vi "log analysis_gps.vi"() -> ()   [LabVIEW 2019] (continued)
-0.0020,-0.483216711,-1.218552457,32.463260828,0.4082,0.2863,0.5249,0.1204,0.1022,0.0792,0.2990,0.3004,4.9651,0f000001,0*7877b410\n\t", "INSPVAXA,USB3,0,45.5,FINESTEERING,2107,281168.650,02000000,471d,15824;INS_ALIGNMENT_COMPLETE,INS_RTKFIXED,37.37019633744,126.72089858847,9.9020,22.3000,0.4572,0.3119,0.0094,-0.439520835,-0.957492339,36.615351128,0.4109,0.2881,0.5277,0.1190,0.0994,0.0787,0.2969,0.2961,4.9653,0f000001,0*c67ea19b\n\t", "INSPVAXA,USB3,0,41.5,FINESTEERING,2107,281169.150,02000000,471d,15824;INS_ALIGNMENT_COMPLETE,INS_RTKFIXED,37.37019803366,126.72090033617,9.8967,22.3000,0.4353,0.3466,-0.0124,-0.373798304,-0.691045943,38.520831977,0.4135,0.2910,0.5324,0.1162,0.0959,0.0784,0.2944,0.2920,4.9653,0f000001,0*85acc37f\n\t", "INSPVAXA,USB3,0,41.5,FINESTEERING,2107,281169.650,02000000,471d,15824;INS_ALIGNMENT_COMPLETE,INS_RTKFIXED,37.37019968370,126.72090219115,9.8910,22.3000,0.4092,0.3296,-0.0191,-0.608129529,-0.998598974,40.257706862,0.4135,0.2910,0.5324,0.1162,0.0959,0.0784,0.2944,0.2920,4.9653,0f000001,0*4e1130ac\n\t", "INSPVAXA,USB3,0,45.5,FINESTEERING,2107,281170.150,02000000,471d,15824;INS_ALIGNMENT_COMPLETE,INS_RTKFIXED,37.37020123427,126.72090408580,9.8830,22.3000,0.3824,0.3449,-0.0045,-0.472006885,-0.997512763,41.710684669,0.4139,0.2909,0.5351,0.1136,0.0932,0.0791,0.2920,0.2885,4.9641,0f000001,0*2dc0ad9b\n\t", "INSPVAXA,USB3,0,45.5,FINESTEERING,2107,281170.650,02000000,471d,15824;INS_ALIGNMENT_COMPLETE,INS_RTKFIXED,37.37020269712,126.72090601410,9.8764,22.3000,0.3826,0.3439,-0.0555,-0.519783559,-1.040179137,42.895943819,0.4139,0.2909,0.5351,0.1136,0.0932,0.0791,0.2920,0.2885,4.9641,0f000001,0*7bedead2\n\t", "INSPVAXA,USB3,0,44.5,FINESTEERING,2107,281171.150,02000000,471d,15824;INS_ALIGNMENT_COMPLETE,INS_RTKFIXED,37.37020410008,126.72090794331,9.8693,22.3000,0.3861,0.3636,0.0003,-0.699793085,-1.013428627,43.781952509,0.4138,0.2914,0.5397,0.1111,0.0916,0.0789,0.2901,0.2864,4.9621,0f000001,0*75d8a529\n\t", "INSPVAXA,USB3,0,44.5,FINESTEERING,2107,281171.650,02000000,471d,15824;INS_ALIGNMENT_COMPLETE,INS_RTKFIXED,37.37020547941,126.72090993032,9.8591,22.3000,0.3712,0.3482,-0.0204,-0.626506310,-1.371933495,44.325085685,0.4138,0.2914,0.5397,0.1111,0.0916,0.0789,0.2901,0.2864,4.9621,0f000001,0*603a8c7d\n\t", "INSPVAXA,USB3,0,46.5,FINESTEERING,2107,281172.150,02000000,471d,15824;INS_ALIGNMENT_COMPLETE,INS_RTKFIXED,37.37020680132,126.72091185634,9.8504,22.3000,0.3423,0.3408,-0.0083,-0.892607382,-1.242115699,44.703288237,0.4137,0.2941,0.5475,0.1101,0.0921,0.0790,0.2889,0.2855,4.9595,0f000001,0*90544be8\n\t", "INSPVAXA,USB3,0,46.5,FINESTEERING,2107,281172.650,02000000,471d,15824;INS_ALIGNMENT_COMPLETE,INS_RTKFIXED,37.37020806274,126.72091379412,9.8428,22.3000,0.3393,0.3608,-0.0229,-0.508945363,-1.293654987,44.950159425,0.4137,0.2941,0.5475,0.1101,0.0921,0.0790,0.2889,0.2855,4.9595,0f000001,0*b56eb890\n\t", "INSPVAXA,USB3,0,45.0,FINESTEERING,2107,281173.150,02000000,471d,15824;INS_ALIGNMENT_COMPLETE,INS_RTKFIXED,37.37020938618,126.72091581251,9.8332,22.3000,0.3324,0.3645,-0.0096,-0.521372580,-0.940346469,45.114108155,0.4131,0.2953,0.5536,0.1104,0.0943,0.0789,0.2883,0.2853,4.9566,0f000001,0*896df924\n\t", "INSPVAXA,USB3,0,45.0,FINESTEERING,2107,281173.650,02000000,471d,15824;INS_ALIGNMENT_COMPLETE,INS_RTKFIXED,37.37021062105,126.72091771518,9.8279,22.3000,0.3141,0.3794,-0.0018,-0.763185421,-1.256731125,45.193767644,0.4131,0.2953,0.5536,0.1104,0.0943,0.0789,0.2883,0.2853,4.9566,0f000001,0*bce21ee6\n\t", "INSPVAXA,USB3,0,42.5,FINESTEERING,2107,281174.150,02000000,471d,15824;INS_ALIGNMENT_COMPLETE,INS_RTKFIXED,37.37021196803,126.72091978453,9.8240,22.3000,0.3107,0.3301,0.0022,-0.763032701,-1.186677441,45.109324656,0.4135,0.2997,0.5622,0.1120,0.0966,0.0795,0.2881,0.2853,4.9521,0f000001,0*4885d5cd\n\t", "INSPVAXA,USB3,0,42.5,FINESTEERING,2107,281174.650,02000000,471d,15824;INS_ALIGNMENT_COMPLETE,INS_RTKFIXED,37.37021324009,126.72092171742,9.8181,22.3000,0.3189,0.3639,-0.0177,-0.623768140,-1.260059850,44.385500285,0.4135,0.2997,0.5622,0.1120,0.0966,0.0795,0.2881,0.2853,4.9521,0f000001,0*5d7db614\n\t", "INSPVAXA,USB3,0,46.0,FINESTEERING,2107,281175.150,02000000,471d,15824;INS_ALIGNMENT_COMPLETE,INS_RTKFIXED,37.37021454485,126.72092359431,9.8111,22.3000,0.2994,0.3285,-0.0007,-0.912779431,-1.090246712,43.056876175,0.4145,0.3032,0.5695,0.1139,0.0990,0.0803,0.2881,0.2850,4.9479,0f000001,0*1b591d65\n\t", "INSPVAXA,USB3,0,46.0,FINESTEERING,2107,281175.650,02000000,471d,15824;INS_ALIGNMENT_COMPLETE,INS_RTKFIXED,37.37021589583,126.72092544139,9.8034,22.3000,0.3183,0.3129,-0.0016,-0.983600306,-1.421345156,41.411365334,0.4145,0.3032,0.5695,0.1139,0.0990,0.0803,0.2881,0.2850,4.9479,0f000001,0*27aaa3ef\n\t", "INSPVAXA,USB3,0,44.5,FINESTEERING,2107,281176.150,02000000,471d,15824;INS_ALIGNMENT_COMPLETE,INS_RTKFIXED,37.37021731136,126.72092726471,9.7967,22.3000,0.3067,0.3205,0.0018,-0.778712195,-1.421988866,39.539976805,0.4163,0.3059,0.5758,0.1149,0.0990,0.0812,0.2880,0.2842,4.9430,0f000001,0*48a96dd4\n\t", "INSPVAXA,USB3,0,44.5,FINESTEERING,2107,281176.650,02000000,471d,15824;INS_ALIGNMENT_COMPLETE,INS_RTKFIXED,37.37021874043,126.72092900172,9.7912,22.3000,0.3343,0.3105,-0.0118,-0.475424413,-1.033048404,37.733219685,0.4163,0.3059,0.5758,0.1149,0.0990,0.0812,0.2880,0.2842,4.9430,0f000001,0*63ca753e\n\t", "INSPVAXA,USB3,0,46.0,FINESTEERING,2107,281177.150,02000000,471d,15824;INS_ALIGNMENT_COMPLETE,INS_RTKFIXED,37.37022027462,126.72093069920,9.7837,22.3000,0.3340,0.3056,-0.0059,-0.436029262,-1.318996825,36.094424232,0.4169,0.3052,0.5779,0.1146,0.0975,0.0816,0.2876,0.2828,4.9395,0f000001,0*8ee0afa4\n\t", "INSPVAXA,USB3,0,46.0,FINESTEERING,2107,281177.650,02000000,471d,15824;INS_ALIGNMENT_COMPLETE,INS_RTKFIXED,37.37022187937,126.72093233106,9.7786,22.3000,0.3383,0.3047,-0.0171,-0.416097585,-1.463260618,34.652814665,0.4169,0.3052,0.5779,0.1146,0.0975,0.0816,0.2876,0.2828,4.9395,0f000001,0*8906ebb7\n\t", "INSPVAXA,USB3,0,43.5,FINESTEERING,2107,281178.150,02000000,471d,15824;INS_ALIGNMENT_COMPLETE,INS_RTKFIXED,37.37022350567,126.72093390601,9.7761,22.3000,0.3475,0.2828,-0.0164,-0.206861779,-1.246508732,33.446442474,0.4170,0.3028,0.5771,0.1137,0.0954,0.0819,0.2871,0.2813,4.9371,0f000001,0*562de2ee\n\t", "INSPVAXA,USB3,0,43.5,FINESTEERING,2107,281178.650,02000000,471d,15824;INS_ALIGNMENT_COMPLETE,INS_RTKFIXED,37.37022519841,126.72093545972,9.7722,22.3000,0.3782,0.2868,-0.0191,-0.115839581,-1.073328137,32.590544637,0.4170,0.3028,0.5771,0.1137,0.0954,0.0819,0.2871,0.2813,4.9371,0f000001,0*73e5bb44\n\t", "INSPVAXA,USB3,0,45.5,FINESTEERING,2107,281179.150,02000000,471d,15824;INS_ALIGNMENT_COMPLETE,INS_RTKFIXED,37.37022690987,126.72093697041,9.7680,22.3000,0.3622,0.2816,-0.0102,-0.207143991,-1.081874423,31.923591302,0.4160,0.2990,0.5741,0.1127,0.0939,0.0821,0.2866,0.2801,4.9362,0f000001,0*5c093e83\n\t", "INSPVAXA,USB3,0,46.5,FINESTEERING,2107,281180.150,02008000,471d,15824;INS_ALIGNMENT_COMPLETE,INS_RTKFIXED,37.37023052669,126.72094007704,9.7564,22.3000,0.3610,0.2647,-0.0164,-0.513272391,-1.387154465,31.645867613,0.4155,0.2970,0.5730,0.1122,0.0935,0.0824,0.2863,0.2794,4.9359,0f000001,0*15d21dba\n\t", "INSPVAXA,USB3,0,46.5,FINESTEERING,2107,281180.650,02008000,471d,15824;INS_ALIGNMENT_COMPLETE,INS_RTKFIXED,37.37023232250,126.72094161397,9.7484,22.3000,0.3885,0.2867,-0.0133,-0.410366705,-1.302704695,31.784927225,0.4155,0.2970,0.5730,0.1122,0.0935,0.0824,0.2863,0.2794,4.9359,0f000001,0*ecf83c2b\n\t", "INSPVAXA,USB3,0,45.5,FINESTEERING,2107,281181.650,02008000,471d,15824;INS_ALIGNMENT_COMPLETE,INS_RTKFIXED,37.37023594976,126.72094471309,9.7312,22.3000,0.3923,0.2955,-0.0276,-0.429360160,-1.491752481,32.266896907,0.4140,0.2923,0.5675,0.1120,0.0932,0.0824,0.2861,0.2791,4.9367,0f000001,0*7730f092\n\t", "INSPVAXA,USB3,0,48.0,FINESTEERING,2107,281183.150,02008000,471d,15824;INS_ALIGNMENT_COMPLETE,INS_RTKFIXED,37.37024155075,126.72094950500,9.7123,22.3000,0.4055,0.2881,-0.0237,-0.200855406,-1.072709947,32.894593043,0.4104,0.2866,0.5571,0.1124,0.0939,0.0825,0.2862,0.2789,4.9396,0f000001,0*f844a638\n\t", "INSPVAXA,USB3,0,49.0,FINESTEERING,2107,281184.650,02008000,471d,15824;INS_ALIGNMENT_COMPLETE,INS_RTKFIXED,37.37024704588,126.72095439123,9.6966,22.3000,0.4339,0.3164,-0.0228,-0.832842396,-1.309145590,33.874103055,0.4098,0.2861,0.5540,0.1127,0.0942,0.0825,0.2862,0.2787,4.9412,0f000001,0*e6c1c908\n\t", "INSPVAXA,USB3,0,44.5,FINESTEERING,2107,281185.650,02008000,471d,15824;INS_ALIGNMENT_COMPLETE,INS_RTKFIXED,37.37025062154,126.72095774565,9.6870,22.3000,0.4074,0.3266,-0.0025,-0.740348806,-1.419761740,34.752841376,0.4093,0.2853,0.5511,0.1123,0.0935,0.0817,0.2862,0.2784,4.9427,0f000001,0*da04eb84\n\t", "INSPVAXA,USB3,0,46.0,FINESTEERING,2107,281186.650,02008000,471d,15824;INS_ALIGNMENT_COMPLETE,INS_RTKFIXED,37.37025416351,126.72096115786,9.6746,22.3000,0.3904,0.3327,-0.0338,-0.811943292,-1.291408071,35.723298207,0.4097,0.2868,0.5516,0.1126,0.0940,0.0823,0.2861,0.2778,4.9442,0f000001,0*aa987070\n\t", "INSPVAXA,USB3,0,42.0,FINESTEERING,2107,281187.150,02008000,471d,15824;INS_ALIGNMENT_COMPLETE,INS_RTKFIXED,37.37025583855,126.72096282892,9.6678,22.3000,0.4091,0.3516,-0.0259,-0.728228198,-1.245007299,36.027390494,0.4101,0.2875,0.5523,0.1126,0.0937,0.0826,0.2859,0.2773,4.9452,0f000001,0*776840fb\n\t", "INSPVAXA,USB3,0,42.5,FINESTEERING,2107,281188.150,02000000,471d,15824;INS_ALIGNMENT_COMPLETE,INS_RTKFIXED,37.37025917986,126.72096621248,9.6609,22.3000,0.4052,0.3240,-0.0181,-0.745275066,-1.101586398,36.822015380,0.4109,0.2894,0.5546,0.1124,0.0934,0.0826,0.2858,0.2767,4.9465,0f000001,0*772ad5b2\n\t", "INSPVAXA,USB3,0,46.5,FINESTEERING,2107,281189.150,02000000,471d,15824;INS_ALIGNMENT_COMPLETE,INS_RTKFIXED,37.37026246505,126.72096957686,9.6575,22.3000,0.3818,0.3519,-0.0175,-0.837192728,-1.183881143,37.353641508,0.4111,0.2898,0.5556,0.1117,0.0925,0.0819,0.2856,0.2763,4.9479,0f000001,0*4984aef6\n\t", "INSPVAXA,USB3,0,47.5,FINESTEERING,2107,281190.150,02000000,471d,15824;INS_ALIGNMENT_COMPLETE,INS_RTKFIXED,37.37026560808,126.72097291937,9.6539,22.3000,0.3854,0.3239,-0.0258,-0.774119778,-1.083116234,37.881716828,0.4108,0.2891,0.5553,0.1117,0.0926,0.0822,0.2854,0.2760,4.9491,0f000001,0*9066855d\n\t", "INSPVAXA,USB3,0,46.5,FINESTEERING,2107,281191.150,02000000,471d,15824;INS_ALIGNMENT_COMPLETE,INS_RTKFIXED,37.37026891266,126.72097643520,9.6441,22.3000,0.4009,0.3345,-0.0087,-0.567088365,-1.086579521,38.077503099,0.4100,0.2882,0.5540,0.1113,0.0920,0.0813,0.2854,0.2758,4.9504,0f000001,0*a8ef7184\n\t", "INSPVAXA,USB3,0,44.5,FINESTEERING,2107,281193.650,02000000,471d,15824;INS_ALIGNMENT_COMPLETE,INS_RTKFIXED,37.37027685595,126.72098468760,9.6314,22.3000,0.3773,0.2845,-0.0187,-0.353904451,-0.860332510,34.629255191,0.4086,0.2861,0.5496,0.1111,0.0919,0.0805,0.2853,0.2756,4.9528,0f000001,0*0c511912\n\t", "INSPVAXA,USB3,0,45.0,FINESTEERING,2107,281195.150,02000000,471d,15824;INS_ALIGNMENT_COMPLETE,INS_RTKFIXED,37.37028195184,126.72098923738,9.6233,22.3000,0.3859,0.2758,0.0067,-0.277560926,-1.244099586,32.051440833,0.4079,0.2838,0.5437,0.1122,0.0928,0.0817,0.2853,0.2754,4.9558,0f000001,0*9827a4c3\n\t", "INSPVAXA,USB3,0,46.0,FINESTEERING,2107,281213.200,02000000,471d,15824;INS_ALIGNMENT_COMPLETE,INS_RTKFIXED,37.37034248828,126.72104733937,9.4372,22.3000,0.3538,0.2828,-0.0066,-0.047417832,-0.921096581,33.030780254,0.4120,0.2924,0.5519,0.1133,0.0939,0.0858,0.2818,0.2696,4.9671,0f000001,0*5574abbc\n\t", "INSPVAXA,USB3,0,45.5,FINESTEERING,2107,281215.200,02000000,471d,15824;INS_ALIGNMENT_COMPLETE,INS_RTKFIXED,37.37034967081,126.72105335114,9.4206,22.3000,0.3913,0.2859,-0.0158,-0.209950038,-1.067150096,30.856231444,0.4131,0.2932,0.5613,0.1129,0.0941,0.0863,0.2814,0.2689,4.9698,0f000001,0*15a1dcfe\n\t", "INSPVAXA,USB3,0,47.5,FINESTEERING,2107,281217.700,02000000,471d,15824;INS_ALIGNMENT_COMPLETE,INS_RTKFIXED,37.37035891275,126.72106070272,9.4027,22.3000,0.3907,0.2751,-0.0370,-0.475151732,-0.956253222,31.086527744,0.4118,0.2907,0.5637,0.1115,0.0927,0.0836,0.2812,0.2687,4.9728,0f000001,0*c5b8ff8b\n\t", "INSPVAXA,USB3,0,41.5,FINESTEERING,2107,281218.700,02000000,471d,15824;INS_ALIGNMENT_COMPLETE,INS_RTKFIXED,37.37036254864,126.72106366487,9.4005,22.3000,0.3951,0.2706,-0.0129,-0.403197852,-0.697835271,31.463679771,0.4109,0.2895,0.5628,0.1119,0.0933,0.0832,0.2811,0.2686,4.9743,0f000001,0*95cb54ca\n\t", "INSPVAXA,USB3,0,45.0,FINESTEERING,2107,281220.700,02000000,471d,15824;INS_ALIGNMENT_COMPLETE,INS_RTKFIXED,37.37036990061,126.72106971349,9.4025,22.3000,0.4109,0.2911,0.0071,-0.800702945,-0.878644990,32.737645043,0.4094,0.2870,0.5571,0.1117,0.0929,0.0807,0.2810,0.2681,4.9772,0f000001,0*67c969e8\n\t", "INSPVAXA,USB3,0,42.5,FINESTEERING,2107,281221.200,02000000,471d,15824;INS_ALIGNMENT_COMPLETE,INS_RTKFIXED,37.37037172466,126.72107126440,9.4031,22.3000,0.4112,0.2890,-0.0190,-0.732165245,-0.750314239,33.130718379,0.4093,0.2853,0.5533,0.1117,0.0926,0.0797,0.2808,0.2678,4.9785,0f000001,0*69bb78c8\n\t", "INSPVAXA,USB3,0,47.0,FINESTEERING,2107,281224.700,02000000,471d,15824;INS_ALIGNMENT_COMPLETE,INS_RTKFIXED,37.37038378890,126.72108266803,9.4041,22.3000,0.3641,0.2986,-0.0101,-0.663611718,-0.597748671,37.087466475,0.4089,0.2830,0.5420,0.1122,0.0925,0.0797,0.2801,0.2667,4.9821,0f000001,0*d2353e58\n\t", "INSPVAXA,USB3,0,49.0,FINESTEERING,2107,281225.700,02008000,471d,15824;INS_ALIGNMENT_COMPLETE,INS_RTKFIXED,37.37038703252,126.72108609198,9.4018,22.3000,0.3794,0.3187,-0.0066,-0.623620259,-0.927536897,37.861250178,0.4087,0.2831,0.5398,0.1124,0.0928,0.0802,0.2799,0.2664,4.9834,0f000001,0*fbb2d3ef\n\t", "INSPVAXA,USB3,0,46.0,FINESTEERING,2107,281226.700,02008000,471d,15824;INS_ALIGNMENT_COMPLETE,INS_RTKFIXED,37.37039019698,126.72108954824,9.4032,22.3000,0.3584,0.3195,-0.0134,-0.717043811,-1.235643045,38.442839555,0.4087,0.2833,0.5380,0.1119,0.0921,0.0796,0.2798,0.2663,4.9847,0f000001,0*b92bfc16\n\t", "INSPVAXA,USB3,0,43.5,FINESTEERING,2107,281227.700,02008000,471d,15824;INS_ALIGNMENT_COMPLETE,INS_RTKFIXED,37.37039325687,126.72109307012,9.3982,22.3000,0.3516,0.3055,0.0005,-0.625802804,-1.271897010,38.869801853,0.4083,0.2827,0.5361,0.1122,0.0924,0.0800,0.2797,0.2662,4.9860,0f000001,0*e8201bda\n\t", "INSPVAXA,USB3,0,44.5,FINESTEERING,2107,281228.200,02008000,471d,15824;INS_ALIGNMENT_COMPLETE,INS_RTKFIXED,37.37039486129,126.72109491850,9.3967,22.3000,0.3668,0.3505,-0.0187,-0.688902140,-1.335982228,38.955777552,0.4076,0.2823,0.5343,0.1119,0.0921,0.0794,0.2796,0.2660,4.9872,0f000001,0*8630753c\n\t", "INSPVAXA,USB3,0,42.5,FINESTEERING,2107,281229.200,02008000,471d,15824;INS_ALIGNMENT_COMPLETE,INS_RTKFIXED,37.37039793167,126.72109852773,9.3953,22.3000,0.3279,0.2928,-0.0255,-0.253376052,-0.991820405,38.455195972,0.4075,0.2825,0.5342,0.1118,0.0921,0.0790,0.2795,0.2658,4.9885,0f000001,0*8eb4cf39\n\t", "INSPVAXA,USB3,0,42.5,FINESTEERING,2107,281229.700,02008000,471d,15824;INS_ALIGNMENT_COMPLETE,INS_RTKFIXED,37.37039951050,126.72110026434,9.3940,22.3000,0.3314,0.2910,-0.0037,-0.337455745,-0.999192864,37.610056402,0.4075,0.2825,0.5342,0.1118,0.0921,0.0790,0.2795,0.2658,4.9885,0f000001,0*825b5af1\n\t", "INSPVAXA,USB3,0,48.0,FINESTEERING,2107,281230.700,02000000,471d,15824;INS_ALIGNMENT_COMPLETE,INS_RTKFIXED,37.37040272369,126.72110367197,9.3887,22.3000,0.3216,0.2986,0.0135,-0.067201953,-1.333373394,35.463092015,0.4076,0.2834,0.5341,0.1119,0.0922,0.0790,0.2794,0.2655,4.9897,0f000001,0*735b730c\n\t", "INSPVAXA,USB3,0,47.0,FINESTEERING,2107,281231.200,02000000,471d,15824;INS_ALIGNMENT_COMPLETE,INS_RTKFIXED,37.37040437272,126.72110529054,9.3853,22.3000,0.3713,0.2903,-0.0029,0.017258070,-1.218794572,34.494374429,0.4079,0.2828,0.5329,0.1115,0.0914,0.0786,0.2791,0.2650,4.9910,0f000001,0*8245b70f\n\t", "INSPVAXA,USB3,0,48.0,FINESTEERING,2107,281232.200,02000000,471d,15824;INS_ALIGNMENT_COMPLETE,INS_RTKFIXED,37.37040781109,126.72110834724,9.3744,22.3000,0.3888,0.2640,-0.0077,-0.124217348,-1.394698716,32.685462252,0.4076,0.2824,0.5319,0.1108,0.0907,0.0781,0.2788,0.2646,4.9925,0f000001,0*3486c657\n\t", "INSPVAXA,USB3,0,48.0,FINESTEERING,2107,281232.700,02000000,471d,15824;INS_ALIGNMENT_COMPLETE,INS_RTKFIXED,37.37040957768,126.72110983569,9.3683,22.3000,0.3693,0.2541,-0.0175,-0.035465033,-1.483738306,31.883679858,0.4076,0.2824,0.5319,0.1108,0.0907,0.0781,0.2788,0.2646,4.9925,0f000001,0*4cf861df\n\t", "INSPVAXA,USB3,0,42.5,FINESTEERING,2107,281233.200,02000000,471d,15824;INS_ALIGNMENT_COMPLETE,INS_RTKFIXED,37.37041136091,126.72111130172,9.3607,22.3000,0.3896,0.2699,-0.0002,0.128694926,-1.559285557,31.391109709,0.4078,0.2816,0.5308,0.1112,0.0913,0.0791,0.2786,0.2642,4.9941,0f000001,0*46ab5c2a\n\t", "INSPVAXA,USB3,0,42.5,FINESTEERING,2107,281233.700,02000000,471d,15824;INS_ALIGNMENT_COMPLETE,INS_RTKFIXED,37.37041314780,126.72111272697,9.3553,22.3000,0.3924,0.2487,-0.0281,0.163758724,-1.359425913,31.096827482,0.4078,0.2816,0.5308,0.1112,0.0913,0.0791,0.2786,0.2642,4.9941,0f000001,0*d64e85f7\n\t", "INSPVAXA,USB3,0,47.0,FINESTEERING,2107,281234.200,02000000,471d,15824;INS_ALIGNMENT_COMPLETE,INS_RTKFIXED,37.37041499218,126.72111417057,9.3481,22.3000,0.4102,0.2507,-0.0208,-0.006261741,-1.350650653,30.806533983,0.4074,0.2813,0.5302,0.1115,0.0918,0.0799,0.2784,0.2639,4.9958,0f000001,0*5fc48718\n\t", "INSPVAXA,USB3,0,47.0,FINESTEERING,2107,281234.700,02000000,471d,15824;INS_ALIGNMENT_COMPLETE,INS_RTKFIXED,37.37041679366,126.72111558413,9.3430,22.3000,0.3853,0.2462,-0.0143,0.055762675,-1.167743160,30.720625161,0.4074,0.2813,0.5302,0.1115,0.0918,0.0799,0.2784,0.2639,4.9958,0f000001,0*9a377d3f\n\t", "INSPVAXA,USB3,0,48.0,FINESTEERING,2107,281235.200,02000000,471d,15824;INS_ALIGNMENT_COMPLETE,INS_RTKFIXED,37.37041862614,126.72111704485,9.3377,22.3000,0.3985,0.2540,-0.0201,0.294289103,-1.099012992,30.736583565,0.4070,0.2811,0.5299,0.1117,0.0922,0.0805,0.2783,0.2638,4.9972,0f000001,0*a95814ac\n\t", "INSPVAXA,USB3,0,44.0,FINESTEERING,2107,281236.200,02000000,471d,15824;INS_ALIGNMENT_COMPLETE,INS_RTKFIXED,37.37042228816,126.72111996191,9.3297,22.3000,0.3967,0.2694,0.0011,0.104811084,-1.415486457,30.958501575,0.4068,0.2811,0.5298,0.1121,0.0927,0.0811,0.2782,0.2636,4.9988,0f000001,0*e69fee41\n\t", "INSPVAXA,USB3,0,44.0,FINESTEERING,2107,281236.700,02000000,471d,15824;INS_ALIGNMENT_COMPLETE,INS_RTKFIXED,37.37042410585,126.72112143606,9.3271,22.3000,0.4148,0.2479,-0.0173,0.069526094,-1.244882003,31.226949687,0.4068,0.2811,0.5298,0.1121,0.0927,0.0811,0.2782,0.2636,4.9988,0f000001,0*974dad1a\n\t", "INSPVAXA,USB3,0,45.5,FINESTEERING,2107,281237.200,02000000,471d,15824;INS_ALIGNMENT_COMPLETE,INS_RTKFIXED,37.37042595037,126.72112294514,9.3228,22.3000,0.4143,0.2621,-0.0195,0.018984845,-1.146574514,31.412832351,0.4068,0.2809,0.5300,0.1124,0.0929,0.0818,0.2782,0.2635,5.0001,0f000001,0*1b0b7511\n\t", "INSPVAXA,USB3,0,46.0,FINESTEERING,2107,281238.200,02000000,471d,15824;INS_ALIGNMENT_COMPLETE,INS_RTKFIXED,37.37042950556,126.72112589522,9.3162,22.3000,0.4227,0.2698,0.0109,-0.200950173,-1.225682197,31.991269010,0.4072,0.2814,0.5306,0.1126,0.0929,0.0821,0.2781,0.2633,5.0015,0f000001,0*0794d365\n\t", "INSPVAXA,USB3,0,46.0,FINESTEERING,2107,281238.700,02000000,471d,15824;INS_ALIGNMENT_COMPLETE,INS_RTKFIXED,37.37043136222,126.72112745012,9.3124,22.3000,0.3943,0.2610,-0.0034,-0.386075100,-1.055396973,32.303525418,0.4072,0.2814,0.5306,0.1126,0.0929,0.0821,0.2781,0.2633,5.0015,0f000001,0*b83f878f\n\t", "INSPVAXA,USB3,0,48.0,FINESTEERING,2107,281239.200,02000000,471d,15824;INS_ALIGNMENT_COMPLETE,INS_RTKFIXED,37.37043317421,126.72112899719,9.3082,22.3000,0.4229,0.2915,-0.0051,-0.601506293,-1.130264131,32.679510223,0.4077,0.2817,0.5313,0.1126,0.0927,0.0822,0.2780,0.2630,5.0030,0f000001,0*20b6ea60\n\t", "INSPVAXA,USB3,0,48.0,FINESTEERING,2107,281239.700,02000000,471d,15824;INS_ALIGNMENT_COMPLETE,INS_RTKFIXED,37.37043494669,126.72113055654,9.3053,22.3000,0.3888,0.2751,0.0114,-0.527038366,-1.080230445,33.250438434,0.4077,0.2817,0.5313,0.1126,0.0927,0.0822,0.2780,0.2630,5.0030,0f000001,0*94791092\n\t", "INSPVAXA,USB3,0,48.5,FINESTEERING,2107,281240.700,02000000,471d,15824;INS_ALIGNMENT_COMPLETE,INS_RTKFIXED,37.37043850253,126.72113379936,9.2976,22.3000,0.4169,0.2904,-0.0141,-0.976451257,-1.265439049,34.098588845,0.4076,0.2813,0.5318,0.1117,0.0919,0.0814,0.2779,0.2627,5.0045,0f000001,0*ee6793dd\n\t", "INSPVAXA,USB3,0,46.5,FINESTEERING,2107,281241.200,02000000,471d,15824;INS_ALIGNMENT_COMPLETE,INS_RTKFIXED,37.37044019660,126.72113544542,9.2926,22.3000,0.4279,0.3108,-0.0036,-0.766553513,-1.370370056,34.585070346,0.4075,0.2803,0.5320,0.1109,0.0908,0.0805,0.2778,0.2623,5.0052,0f000001,0*260ccca0\n\t", "INSPVAXA,USB3,0,46.5,FINESTEERING,2107,281241.700,02000000,471d,15824;INS_ALIGNMENT_COMPLETE,INS_RTKFIXED,37.37044183342,126.72113705465,9.2914,22.3000,0.3729,0.2861,0.0243,-0.736192584,-1.169550873,35.066959350,0.4075,0.2803,0.5320,0.1109,0.0908,0.0805,0.2778,0.2623,5.0052,0f000001,0*7de3fdbf\n\t", "INSPVAXA,USB3,0,46.5,FINESTEERING,2107,281242.200,02000000,471d,15824;INS_ALIGNMENT_COMPLETE,INS_RTKFIXED,37.37044357732,126.72113877934,9.2913,22.3000,0.3995,0.2989,-0.0112,-0.773150570,-1.240971766,35.457586747,0.4072,0.2799,0.5319,0.1103,0.0904,0.0797,0.2776,0.2620,5.0062,0f000001,0*047104d0\n\t", "INSPVAXA,USB3,0,46.5,FINESTEERING,2107,281242.700,02000000,471d,15824;INS_ALIGNMENT_COMPLETE,INS_RTKFIXED,37.37044518884,126.72114042326,9.2923,22.3000,0.3596,0.3049,0.0120,-0.827179513,-0.912103368,35.739029632,0.4072,0.2799,0.5319,0.1103,0.0904,0.0797,0.2776,0.2620,5.0062,0f000001,0*089314b8\n\t", "INSPVAXA,USB3,0,47.5,FINESTEERING,2107,281243.200,02000000,471d,15824;INS_ALIGNMENT_COMPLETE,INS_RTKFIXED,37.37044682347,126.72114212345,9.2944,22.3000,0.3805,0.3012,0.0098,-0.728489494,-1.051472192,36.148202459,0.4069,0.2798,0.5321,0.1112,0.0916,0.0809,0.2775,0.2618,5.0071,0f000001,0*ab715168\n\t", "INSPVAXA,USB3,0,47.5,FINESTEERING,2107,281243.700,02000000,471d,15824;INS_ALIGNMENT_COMPLETE,INS_RTKFIXED,37.37044842257,126.72114379217,9.2929,22.3000,0.3497,0.2949,0.0009,-0.706502684,-0.959221575,36.485073335,0.4069,0.2798,0.5321,0.1112,0.0916,0.0809,0.2775,0.2618,5.0071,0f000001,0*0606f155\n\t", "INSPVAXA,USB3,0,48.0,FINESTEERING,2107,281244.200,02000000,471d,15824;INS_ALIGNMENT_COMPLETE,INS_RTKFIXED,37.37045000855,126.72114549963,9.2935,22.3000,0.3813,0.3173,-0.0073,-0.659947391,-1.102241434,36.768615727,0.4069,0.2807,0.5325,0.1118,0.0924,0.0817,0.2773,0.2617,5.0086,0f000001,0*dffaeeda\n\t", "INSPVAXA,USB3,0,48.0,FINESTEERING,2107,281244.700,02000000,471d,15824;INS_ALIGNMENT_COMPLETE,INS_RTKFIXED,37.37045160181,126.72114725109,9.2936,22.3000,0.3610,0.3198,-0.0165,-0.651308584,-1.162087576,36.974039680,0.4069,0.2807,0.5325,0.1118,0.0924,0.0817,0.2773,0.2617,5.0086,0f000001,0*f70d22ce\n\t", "INSPVAXA,USB3,0,45.5,FINESTEERING,2107,281245.200,02000000,471d,15824;INS_ALIGNMENT_COMPLETE,INS_RTKFIXED,37.37045318824,126.72114900963,9.2932,22.3000,0.3383,0.3092,0.0249,-0.721431516,-1.066505457,37.188586073,0.4071,0.2814,0.5325,0.1122,0.0928,0.0822,0.2772,0.2616,5.0103,0f000001,0*ccafe7f7\n\t", "INSPVAXA,USB3,0,45.5,FINESTEERING,2107,281245.700,02000000,471d,15824;INS_ALIGNMENT_COMPLETE,INS_RTKFIXED,37.37045471115,126.72115068638,9.2913,22.3000,0.3729,0.3102,-0.0028,-0.841928711,-1.027529391,37.390122228,0.4071,0.2814,0.5325,0.1122,0.0928,0.0822,0.2772,0.2616,5.0103,0f000001,0*6bbac107\n\t", "INSPVAXA,USB3,0,45.5,FINESTEERING,2107,281246.200,02000000,471d,15824;INS_ALIGNMENT_COMPLETE,INS_RTKFIXED,37.37045637770,126.72115252290,9.2880,22.3000,0.3686,0.3330,-0.0134,-0.785462216,-0.911426514,37.597924060,0.4074,0.2823,0.5331,0.1123,0.0929,0.0823,0.2772,0.2616,5.0118,0f000001,0*adb8b62a\n\t", "INSPVAXA,USB3,0,45.5,FINESTEERING,2107,281246.700,02000000,471d,15824;INS_ALIGNMENT_COMPLETE,INS_RTKFIXED,37.37045798543,126.72115430749,9.2870,22.3000,0.3687,0.3323,0.0184,-0.822794799,-1.314908192,37.714000338,0.4074,0.2823,0.5331,0.1123,0.0929,0.0823,0.2772,0.2616,5.0118,0f000001,0*e142e69f\n\t", "INSPVAXA,USB3,0,47.0,FINESTEERING,2107,281247.200,02000000,471d,15824;INS_ALIGNMENT_COMPLETE,INS_RTKFIXED,37.37045959180,126.72115606878,9.2846,22.3000,0.3414,0.3044,0.0046,-0.926007496,-1.283685718,37.475312955,0.4073,0.2824,0.5333,0.1125,0.0929,0.0824,0.2771,0.2615,5.0133,0f000001,0*cd9ecdd0\n\t", "INSPVAXA,USB3,0,47.0,FINESTEERING,2107,281247.700,02000000,471d,15824;INS_ALIGNMENT_COMPLETE,INS_RTKFIXED,37.37046119890,126.72115783063,9.2839,22.3000,0.3362,0.3158,0.0008,-0.640262260,-1.260973673,36.963677564,0.4073,0.2824,0.5333,0.1125,0.0929,0.0824,0.2771,0.2615,5.0133,0f000001,0*29beb2b2\n\t", "INSPVAXA,USB3,0,44.5,FINESTEERING,2107,281248.200,02000000,471d,15824;INS_ALIGNMENT_COMPLETE,INS_RTKFIXED,37.37046280365,126.72115953545,9.2819,22.3000,0.3356,0.2942,0.0022,-0.584668028,-1.162399511,36.175550915,0.4076,0.2828,0.5341,0.1126,0.0930,0.0826,0.2771,0.2613,5.0149,0f000001,0*7d42a3a6\n\t", "INSPVAXA,USB3,0,44.5,FINESTEERING,2107,281248.700,02000000,471d,15824;INS_ALIGNMENT_COMPLETE,INS_RTKFIXED,37.37046444744,126.72116118616,9.2798,22.3000,0.3405,0.3106,0.0054,-0.632258383,-1.342162283,35.326473382,0.4076,0.2828,0.5341,0.1126,0.0930,0.0826,0.2771,0.2613,5.0149,0f000001,0*74672090\n\t", "INSPVAXA,USB3,0,47.0,FINESTEERING,2107,281249.200,02000000,471d,15824;INS_ALIGNMENT_COMPLETE,INS_RTKFIXED,37.37046613756,126.72116281120,9.2778,22.3000,0.3636,0.2914,-0.0245,-0.793213759,-1.308005739,34.279375865,0.4077,0.2829,0.5343,0.1125,0.0927,0.0827,0.2770,0.2611,5.0165,0f000001,0*423f42ab\n\t", "INSPVAXA,USB3,0,47.0,FINESTEERING,2107,281249.700,02000000,471d,15824;INS_ALIGNMENT_COMPLETE,INS_RTKFIXED,37.37046782429,126.72116439837,9.2744,22.3000,0.3684,0.2690,0.0171,-0.693439264,-1.326725585,33.382125855,0.4077,0.2829,0.5343,0.1125,0.0927,0.0827,0.2770,0.2611,5.0165,0f000001,0*88d26f4b\n\t", "INSPVAXA,USB3,0,48.5,FINESTEERING,2107,281250.200,02000000,471d,15824;INS_ALIGNMENT_COMPLETE,INS_RTKFIXED,37.37046951993,126.72116592037,9.2722,22.3000,0.3585,0.2583,-0.0083,-0.676233925,-1.068835400,32.415403285,0.4082,0.2827,0.5347,0.1117,0.0917,0.0817,0.2769,0.2609,5.0181,0f000001,0*23e1d120\n\t", "INSPVAXA,USB3,0,48.5,FINESTEERING,2107,281250.700,02000000,471d,15824;INS_ALIGNMENT_COMPLETE,INS_RTKFIXED,37.37047125659,126.72116740651,9.2700,22.3000,0.3759,0.2852,-0.0005,-0.704418512,-1.024345278,31.769899431,0.4082,0.2827,0.5347,0.1117,0.0917,0.0817,0.2769,0.2609,5.0181,0f000001,0*220f1c57\n\t", "INSPVAXA,USB3,0,46.0,FINESTEERING,2107,281251.200,02000000,471d,15824;INS_ALIGNMENT_COMPLETE,INS_RTKFIXED,37.37047303421,126.72116889318,9.2673,22.3000,0.3786,0.2715,-0.0144,-0.713801343,-0.929392253,31.230715731,0.4077,0.2824,0.5344,0.1113,0.0913,0.0813,0.2767,0.2607,5.0197,0f000001,0*81e3f7b1\n\t", "INSPVAXA,USB3,0,46.0,FINESTEERING,2107,281251.700,02000000,471d,15824;INS_ALIGNMENT_COMPLETE,INS_RTKFIXED,37.37047481505,126.72117034620,9.2660,22.3000,0.4016,0.2734,-0.0090,-0.658846991,-1.106608605,30.760952278,0.4077,0.2824,0.5344,0.1113,0.0913,0.0813,0.2767,0.2607,5.0197,0f000001,0*148382ef\n\t", "DUALANTENNAHEADINGA,USB3,0,47.5,FINESTEERING,2107,281252.200,02000000,d426,15824;SOL_COMPUTED,NARROW_INT,-1.000000000,33.188526154,-13.188842773,0.0,2.061341047,2.951399803,\"631T\",23,11,11,8,04,00,30,03*cb8882ef\n\t", "INSPVAXA,USB3,0,47.5,FINESTEERING,2107,281252.700,02000000,471d,15824;INS_ALIGNMENT_COMPLETE,INS_RTKFIXED,37.37047843924,126.72117325955,9.2610,22.3000,0.3921,0.2613,-0.0047,-0.684255773,-1.075453896,30.582940759,0.4074,0.2818,0.5338,0.1112,0.0914,0.0811,0.2766,0.2605,5.0213,0f000001,0*2a48569e\n\t", "INSPVAXA,USB3,0,43.0,FINESTEERING,2107,281253.200,02000000,471d,15824;INS_ALIGNMENT_COMPLETE,INS_RTKFIXED,37.37048028352,126.72117473138,9.2588,22.3000,0.4035,0.2637,-0.0100,-0.810109039,-1.254597074,30.636904174,0.4069,0.2810,0.5332,0.1116,0.0919,0.0813,0.2766,0.2604,5.0230,0f000001,0*5ad017a3\n\t", "INSPVAXA,USB3,0,43.0,FINESTEERING,2107,281253.700,02000000,471d,15824;INS_ALIGNMENT_COMPLETE,INS_RTKFIXED,37.37048209975,126.72117619764,9.2563,22.3000,0.3713,0.2637,0.0057,-0.851136765,-1.427746599,30.748659143,0.4069,0.2810,0.5332,0.1116,0.0919,0.0813,0.2766,0.2604,5.0230,0f000001,0*3581eb98\n\t", "INSPVAXA,USB3,0,41.5,FINESTEERING,2107,281254.200,02000000,471d,15824;INS_ALIGNMENT_COMPLETE,INS_RTKFIXED,37.37048389322,126.72117766049,9.2543,22.3000,0.4011,0.2685,-0.0017,-0.904192173,-1.398090908,30.961508821,0.4078,0.2816,0.5344,0.1121,0.0926,0.0815,0.2766,0.2603,5.0245,0f000001,0*1f3e2204\n\t", "INSPVAXA,USB3,0,41.5,FINESTEERING,2107,281254.700,02000000,471d,15824;INS_ALIGNMENT_COMPLETE,INS_RTKFIXED,37.37048568888,126.72117913940,9.2511,22.3000,0.3906,0.2712,-0.0003,-0.736378348,-1.044906889,31.224322572,0.4078,0.2816,0.5344,0.1121,0.0926,0.0815,0.2766,0.2603,5.0245,0f000001,0*c5f145ca\n\t", "INSPVAXA,USB3,0,44.0,FINESTEERING,2107,281255.200,02000000,471d,15824;INS_ALIGNMENT_COMPLETE,INS_RTKFIXED,37.37048748822,126.72118062065,9.2468,22.3000,0.4035,0.2848,0.0108,-0.751779766,-1.053207928,31.437162852,0.4105,0.2861,0.5416,0.1127,0.0935,0.0821,0.2766,0.2602,5.0258,0f000001,0*b06b1cec\n\t", "INSPVAXA,USB3,0,44.0,FINESTEERING,2107,281255.700,02000000,471d,15824;INS_ALIGNMENT_COMPLETE,INS_RTKFIXED,37.37048934103,126.72118213039,9.2433,22.3000,0.4087,0.2855,0.0141,-0.905392438,-1.018943356,31.720261979,0.4105,0.2861,0.5416,0.1127,0.0935,0.0821,0.2766,0.2602,5.0258,0f000001,0*e5e8b97b\n\t", "INSPVAXA,USB3,0,48.5,FINESTEERING,2107,281256.200,02000000,471d,15824;INS_ALIGNMENT_COMPLETE,INS_RTKFIXED,37.37049116166,126.72118365474,9.2406,22.3000,0.4005,0.2755,-0.0046,-0.741933390,-0.975317507,31.970856097,0.4116,0.2891,0.5469,0.1124,0.0932,0.0816,0.2765,0.2599,5.0273,0f000001,0*39271fda\n\t", "INSPVAXA,USB3,0,48.5,FINESTEERING,2107,281256.700,02000000,471d,15824;INS_ALIGNMENT_COMPLETE,INS_RTKFIXED,37.37049294777,126.72118517063,9.2381,22.3000,0.3986,0.2835,-0.0013,-0.674369824,-1.134847367,32.198409844,0.4116,0.2891,0.5469,0.1124,0.0932,0.0816,0.2765,0.2599,5.0273,0f000001,0*38bc1ccb\n\t", "INSPVAXA,USB3,0,42.5,FINESTEERING,2107,281257.200,02000000,471d,15824;INS_ALIGNMENT_COMPLETE,INS_RTKFIXED,37.37049476461,126.72118674012,9.2353,22.3000,0.4039,0.2899,0.0228,-0.674986322,-0.804758073,32.620444545,0.4119,0.2902,0.5497,0.1119,0.0926,0.0809,0.2764,0.2596,5.0289,0f000001,0*72dede25\n\t", "DUALANTENNAHEADINGA,USB3,0,42.5,FINESTEERING,2107,281257.700,02000000,d426,15824;SOL_COMPUTED,NARROW_INT,-1.000000000,35.851467133,-13.614562988,0.0,0.761796772,1.619968295,\"631T\",20,13,13,10,04,00,30,33*8335f7c7\n\t", "DUALANTENNAHEADINGA,USB3,0,50.0,FINESTEERING,2107,281258.200,02000000,d426,15824;SOL_COMPUTED,NARROW_INT,-1.000000000,36.208633423,-13.477111816,0.0,0.769826293,1.626826406,\"631T\",21,13,13,10,04,00,30,33*663662cf\n\t", "DUALANTENNAHEADINGA,USB3,0,50.0,FINESTEERING,2107,281258.700,02000000,d426,15824;SOL_COMPUTED,NARROW_INT,-1.000000000,37.583648682,-15.574401855,0.0,0.757817268,1.584750891,\"631T\",22,13,13,10,04,00,30,33*2671cfe0\n\t", "INSPVAXA,USB3,0,44.5,FINESTEERING,2107,281259.200,02000000,471d,15824;INS_ALIGNMENT_COMPLETE,INS_RTKFIXED,37.37050172881,126.72119309205,9.2293,22.3000,0.3645,0.2781,0.0053,-0.664590657,-1.103713757,34.708593103,0.4125,0.2928,0.5558,0.1115,0.0923,0.0801,0.2762,0.2590,5.0316,0f000001,0*10acd44c\n\t", "DUALANTENNAHEADINGA,USB3,0,44.5,FINESTEERING,2107,281259.700,02000000,d426,15824;SOL_COMPUTED,NARROW_INT,-1.000000000,37.724102020,-13.091491699,0.0,0.801039636,1.911924362,\"631T\",23,13,13,10,04,00,30,33*9a10e697\n\t", "DUALANTENNAHEADINGA,USB3,0,46.0,FINESTEERING,2107,281260.200,02000000,d426,15824;SOL_COMPUTED,NARROW_INT,-1.000000000,39.115306854,-14.136718750,0.0,0.803064227,1.840907216,\"631T\",22,13,13,10,04,00,30,33*b50651c8\n\t", "INSPVAXA,USB3,0,46.0,FINESTEERING,2107,281260.700,02000000,471d,15824;INS_ALIGNMENT_COMPLETE,INS_RTKFIXED,37.37050659731,126.72119803894,9.2129,22.3000,0.3476,0.2954,-0.0046,-0.736337241,-0.866215786,36.967370061,0.4129,0.2931,0.5580,0.1111,0.0922,0.0796,0.2761,0.2587,5.0324,0f000001,0*f680867e\n\t", "DUALANTENNAHEADINGA,USB3,0,47.0,FINESTEERING,2107,281261.200,02000000,d426,15824;SOL_COMPUTED,NARROW_INT,-1.000000000,40.638893127,-14.791442871,0.0,0.948415875,1.839464903,\"631T\",22,13,13,10,04,00,30,33*e03d9ee2\n\t", "DUALANTENNAHEADINGA,USB3,0,47.0,FINESTEERING,2107,281261.700,02000000,d426,15824;SOL_COMPUTED,NARROW_INT,-1.000000000,41.109539032,-15.221740723,0.0,0.905525208,1.730005383,\"631T\",23,13,13,10,04,00,30,33*024d4917\n\t", "INSPVAXA,USB3,0,48.5,FINESTEERING,2107,281262.200,02000000,471d,15824;INS_ALIGNMENT_COMPLETE,INS_RTKFIXED,37.37051135322,126.72120322169,9.1946,22.3000,0.3493,0.3226,-0.0187,-1.003564380,-0.949445467,38.532803613,0.4120,0.2907,0.5583,0.1108,0.0918,0.0785,0.2758,0.2584,5.0341,0f000001,0*bc77f761\n\t", "DUALANTENNAHEADINGA,USB3,0,48.5,FINESTEERING,2107,281262.700,02000000,d426,15824;SOL_COMPUTED,NARROW_INT,-1.000000000,41.024471283,-13.771057129,0.0,0.941205680,1.970374942,\"631T\",22,13,13,10,04,00,30,33*2b107b4d\n\t", "INSPVAXA,USB3,0,45.5,FINESTEERING,2107,281263.200,02000000,471d,15824;INS_ALIGNMENT_COMPLETE,INS_RTKFIXED,37.37051438675,126.72120667905,9.1791,22.3000,0.3385,0.3277,0.0132,-0.749117776,-1.036053021,39.114622535,0.4097,0.2867,0.5508,0.1108,0.0917,0.0777,0.2757,0.2582,5.0350,0f000001,0*900f5f81\n\t", "INSPVAXA,USB3,0,45.5,FINESTEERING,2107,281263.700,02000000,471d,15824;INS_ALIGNMENT_COMPLETE,INS_RTKFIXED,37.37051592724,126.72120843066,9.1725,22.3000,0.3345,0.3100,-0.0269,-0.953062315,-1.001119813,39.367076268,0.4097,0.2867,0.5508,0.1108,0.0917,0.0777,0.2757,0.2582,5.0350,0f000001,0*3f1ff118\n\t", "DUALANTENNAHEADINGA,USB3,0,45.5,FINESTEERING,2107,281264.200,02000000,d426,15824;SOL_COMPUTED,NARROW_INT,-1.000000000,41.910186768,-13.638671875,0.0,0.987370729,2.013862848,\"631T\",24,13,13,10,04,00,30,33*886cbc18\n\t", "DUALANTENNAHEADINGA,USB3,0,45.5,FINESTEERING,2107,281264.700,02000000,d426,15824;SOL_COMPUTED,NARROW_INT,-1.000000000,42.165882111,-13.191467285,0.0,1.231637120,2.283805132,\"631T\",23,11,11,8,04,00,30,03*d347cf5b\n\t", "DUALANTENNAHEADINGA,USB3,0,48.5,FINESTEERING,2107,281265.200,02000000,d426,15824;SOL_COMPUTED,NARROW_INT,-1.000000000,41.782566071,-14.026184082,0.0,0.949394464,1.456767678,\"631T\",24,12,12,8,04,00,30,03*b5e68f03\n\t", "DUALANTENNAHEADINGA,USB3,0,48.5,FINESTEERING,2107,281265.700,02000000,d426,15824;SOL_COMPUTED,NARROW_INT,-1.000000000,42.654987335,-13.940582275,0.0,0.905997872,1.456194401,\"631T\",25,12,12,8,04,00,30,03*ebbb69a1\n\t", "DUALANTENNAHEADINGA,USB3,0,44.0,FINESTEERING,2107,281266.200,02000000,d426,15824;SOL_COMPUTED,NARROW_INT,-1.000000000,41.473289490,-13.976562500,0.0,0.876108646,1.437642574,\"631T\",26,12,12,8,04,00,30,03*9c4cfbf2\n\t", "INSPVAXA,USB3,0,44.0,FINESTEERING,2107,281266.700,02000000,471d,15824;INS_ALIGNMENT_COMPLETE,INS_RTKFIXED,37.37052514721,126.72121924696,9.1351,22.3000,0.3260,0.3161,-0.0126,-0.947375074,-0.706024295,38.522505124,0.4363,0.2885,0.5509,0.1172,0.0950,0.0803,0.2752,0.2577,5.0353,0f000001,0*ab36857c\n\t", "DUALANTENNAHEADINGA,USB3,0,48.0,FINESTEERING,2107,281267.200,02000000,d426,15824;SOL_COMPUTED,NARROW_INT,-1.000000000,40.023796082,-13.769653320,0.0,1.105050921,2.107353687,\"631T\",22,12,12,8,04,00,30,03*89f55c6d\n\t", "DUALANTENNAHEADINGA,USB3,0,48.0,FINESTEERING,2107,281267.700,02000000,d426,15824;SOL_COMPUTED,NARROW_INT,-1.000000000,38.975990295,-14.866943359,0.0,1.019285679,1.869416475,\"631T\",22,12,12,8,04,00,30,03*a0488b34\n\t", "DUALANTENNAHEADINGA,USB3,0,48.0,FINESTEERING,2107,281268.200,02000000,d426,15824;SOL_COMPUTED,NARROW_INT,-1.000000000,37.457145691,-14.142669678,0.0,0.916966915,1.645377994,\"631T\",25,12,12,8,04,00,30,03*51ae3b94\n\t", "DUALANTENNAHEADINGA,USB3,0,48.0,FINESTEERING,2107,281268.700,02000000,d426,15824;SOL_COMPUTED,NARROW_INT,-1.000000000,36.570995331,-12.889495850,0.0,0.874405205,1.610776067,\"631T\",27,12,12,8,04,00,30,03*59172eb5\n\t", "DUALANTENNAHEADINGA,USB3,0,43.5,FINESTEERING,2107,281269.200,02000000,d426,15824;SOL_COMPUTED,NARROW_INT,-1.000000000,35.973979950,-14.332061768,0.0,0.830094159,1.497864485,\"631T\",27,12,12,8,04,00,30,03*090ddc0d\n\t", "DUALANTENNAHEADINGA,USB3,0,43.5,FINESTEERING,2107,281269.700,02000000,d426,15824;SOL_COMPUTED,NARROW_INT,-1.000000000,35.818984985,-16.138092041,0.0,0.812042832,1.471114397,\"631T\",26,12,12,8,04,00,30,03*f4bb3c31\n\t", "DUALANTENNAHEADINGA,USB3,0,46.5,FINESTEERING,2107,281270.200,02000000,d426,15824;SOL_COMPUTED,NARROW_INT,-1.000000000,35.621791840,-13.436737061,0.0,0.778346181,1.418952346,\"631T\",25,12,12,8,04,00,30,03*c6e6dbb2\n\t", "DUALANTENNAHEADINGA,USB3,0,46.5,FINESTEERING,2107,281270.700,02000000,d426,15824;SOL_COMPUTED,NARROW_INT,-1.000000000,35.070240021,-13.728149414,0.0,0.744003534,1.356679201,\"631T\",25,12,12,8,04,00,30,03*cf10d1c9\n\t", "DUALANTENNAHEADINGA,USB3,0,45.5,FINESTEERING,2107,281271.200,02000000,d426,15824;SOL_COMPUTED,NARROW_INT,-1.000000000,35.494377136,-13.422943115,0.0,0.983616889,2.186612129,\"631T\",23,12,12,8,04,00,30,03*afbd86f5\n\t", "DUALANTENNAHEADINGA,USB3,0,45.5,FINESTEERING,2107,281271.700,02000000,d426,15824;SOL_COMPUTED,NARROW_INT,-1.000000000,35.115871429,-12.229492188,0.0,0.917624831,2.129554033,\"631T\",22,11,11,8,04,00,30,03*47d1ca67\n\t", "DUALANTENNAHEADINGA,USB3,0,45.0,FINESTEERING,2107,281272.200,02000000,d426,15824;SOL_COMPUTED,NARROW_INT,-1.000000000,35.165107727,-13.680572510,0.0,0.853601813,1.895400286,\"631T\",23,11,11,8,04,00,30,03*664b8012\n\t", "DUALANTENNAHEADINGA,USB3,0,45.0,FINESTEERING,2107,281272.700,02000000,d426,15824;SOL_COMPUTED,NARROW_INT,-1.000000000,35.308296204,-13.433410645,0.0,0.833106577,1.789978504,\"631T\",23,11,11,8,04,00,30,03*efeaf6da\n\t", "DUALANTENNAHEADINGA,USB3,0,46.0,FINESTEERING,2107,281273.200,02000000,d426,15824;SOL_COMPUTED,NARROW_INT,-1.000000000,36.192741394,-16.037811279,0.0,0.810550869,1.694264531,\"631T\",22,11,11,8,04,00,30,03*4456d48d\n\t", "DUALANTENNAHEADINGA,USB3,0,48.0,FINESTEERING,2107,281274.200,02000000,d426,15824;SOL_COMPUTED,NARROW_INT,-1.000000000,35.622310638,-14.246795654,0.0,1.186534643,2.124257803,\"631T\",23,13,13,10,04,00,30,33*4699dedc\n\t", "DUALANTENNAHEADINGA,USB3,0,45.0,FINESTEERING,2107,281275.200,02000000,d426,15824;SOL_COMPUTED,NARROW_INT,-1.000000000,35.922065735,-12.943084717,0.0,1.068319321,2.159161329,\"631T\",24,13,13,10,04,00,30,23*90535b08\n\t", "DUALANTENNAHEADINGA,USB3,0,45.0,FINESTEERING,2107,281275.700,02000000,d426,15824;SOL_COMPUTED,NARROW_INT,-1.000000000,35.806697845,-14.127471924,0.0,1.191707134,2.929863453,\"631T\",23,13,13,10,04,00,30,33*14f638f6\n\t", "DUALANTENNAHEADINGA,USB3,0,47.5,FINESTEERING,2107,281277.200,02000000,d426,15824;SOL_COMPUTED,NARROW_INT,-1.000000000,36.727424622,-13.082946777,0.0,0.949807763,2.157425642,\"631T\",23,11,11,8,04,00,30,03*dbda4352\n\t", "DUALANTENNAHEADINGA,USB3,0,47.0,FINESTEERING,2107,281278.200,02000000,d426,15824;SOL_COMPUTED,NARROW_INT,-1.000000000,38.801025391,-13.665405273,0.0,1.011600971,2.213801622,\"631T\",23,11,11,8,04,00,30,03*a2b4300d\n\t", "DUALANTENNAHEADINGA,USB3,0,44.5,FINESTEERING,2107,281279.200,02000000,d426,15824;SOL_COMPUTED,NARROW_INT,-1.000000000,39.271907806,-13.744201660,0.0,0.885574758,1.866288543,\"631T\",24,11,11,8,04,00,30,03*14651a74\n\t", "DUALANTENNAHEADINGA,USB3,0,48.0,FINESTEERING,2107,281280.700,02000000,d426,15824;SOL_COMPUTED,NARROW_INT,-1.000000000,40.700374603,-12.203552246,0.0,0.796584129,1.643284798,\"631T\",24,11,11,8,04,00,30,03*0355bfc3\n\t", "DUALANTENNAHEADINGA,USB3,0,43.5,FINESTEERING,2107,281281.700,02000000,d426,15824;SOL_COMPUTED,NARROW_INT,-1.000000000,41.025180817,-13.610565186,0.0,1.006764770,1.762146711,\"631T\",23,11,11,8,04,00,30,03*95eb9222\n\t", "DUALANTENNAHEADINGA,USB3,0,48.5,FINESTEERING,2107,281282.700,02000000,d426,15824;SOL_COMPUTED,NARROW_INT,-1.000000000,42.471115112,-14.988128662,0.0,1.268621087,2.738634586,\"631T\",23,13,13,9,04,00,20,23*7676e672\n\t", "INSPVAXA,USB3,0,48.0,FINESTEERING,2107,281283.250,02000000,471d,15824;INS_ALIGNMENT_COMPLETE,INS_RTKFIXED,37.37058125614,126.72127316558,9.0365,22.3000,0.3478,0.3335,-0.0027,-0.704403404,-0.836236554,39.118701803,0.4319,0.3133,0.6216,0.1204,0.1024,0.0974,0.2734,0.2534,5.0561,0f000001,0*0df7e601\n\t", "DUALANTENNAHEADINGA,USB3,0,48.0,FINESTEERING,2107,281283.700,02000000,d426,15824;SOL_COMPUTED,NARROW_INT,-1.000000000,
